vi "Create Data Channels.vi"(8 "error in":errorcluster, 11 "Node in":refnum<class "AMS Power Supply Template.lvclass">) -> (0 "error out":errorcluster, 3 "Node out":refnum<class "AMS Power Supply Template.lvclass">)   [LabVIEW 2023, in "AMS Power Supply Template.lvlib" / "AMS Power Supply Template.lvclass"]
uses:
  AMS Power Supply Template.lvclass
  C:/Program Files/National Instruments/LabVIEW 2024/vi.lib/ADAS Replay HIL/Template Node/Plugin/Template Node/Template Node.lvclass
  <vilib>/ADAS Replay HIL/Template Node/Plugin/Template Node/Template Node.lvclass/Template Node.ctl
  AMS Power Supply Template.lvclass/AMS Power Supply Template.ctl
  C:/Program Files/National Instruments/BLS plugin/Capabilities/Capabilities/High Level Capabilities/Power Supply/Power Supply.lvclass
  <vilib>/ADAS Replay HIL/Template Node/Plugin/Template Node/Template Node.lvclass
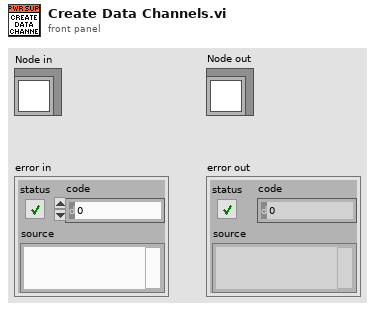
[diagram p1: front panel]
types:
  T1 = typedef "AMS Power Supply Template.lvlib/AMS Power Supply Template.lvclass/Configuration Params.ctl" = cluster{"Common":T2, "Amount of Channels":u32, "Address":string}
  T2 = typedef "Template Node.lvlib/Template Node.lvclass/Common Configuration Params.ctl" = cluster{"Iteration Interval (s)":dbl, "T0 (ns)":u64, "Priority":i32, "Processor":i32, "Wait in Ready State":bool}
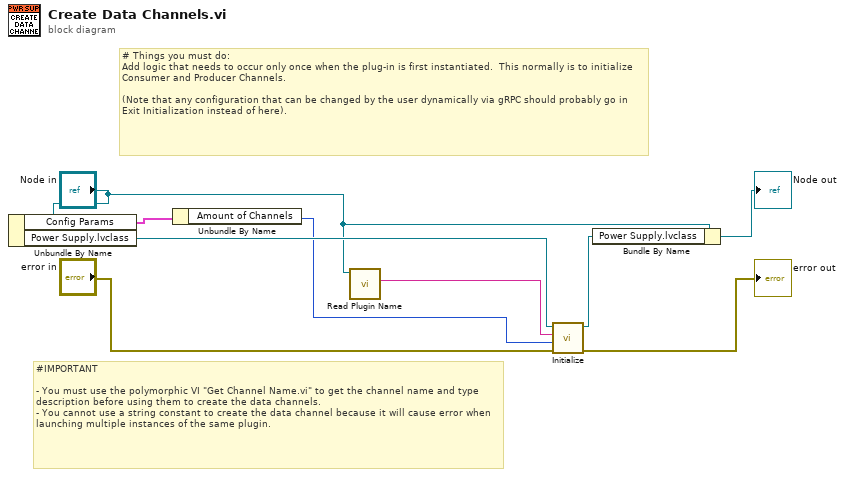
[diagram p0: block diagram]
diagram:
  # "# Things you must do:\nAdd logic that needs to occur only once when the plug-in is first instantiated.  This normally is to initialize Consumer and Producer Channels.   \n\n(Note that any configuration that can be changed by the user dynamically via gRPC should probably go in Exit Initialization instead of here)."
  # "#IMPORTANT\n\n- You must use the polymorphic VI \"Get Channel Name.vi\" to get the channel name and type description before using them to create the data channels.\n- You cannot use a string constant to create the data channel because it will cause error when launching multiple instances of the same plugin."
  n1 = Unbundle By Name("Node in") -> ("Config Params"=w2:T1, "Power Supply.lvclass"=w4:refnum<class "Power Supply.lvclass">)
  n2 = Unbundle By Name(w2) -> ("Amount of Channels"=w1:u32)
  n3 = call <vilib>:"Read Plugin Name.vi"("Template Node in"="Node in") -> ("Plugin Name"=w7:string)  [unwired: 8 in, 2 out]
  n4 = call-dynamic "Initialize.vi"("error in"="error in", "Number of Channels"=w1, "Instance Name"=w7, "Power Supply In"=w4) -> ("error out"=→"error out":errorcluster, "Power Supply Out"=w5:refnum<class "Power Supply.lvclass">)  [unwired: 6 in]
  n5 = Bundle By Name(cluster="Node in", "Power Supply.lvclass"=w5) -> (→"Node out":refnum<class "AMS Power Supply Template.lvclass">)
